vi "ChangeIndicator_RT.vi"(0 "Input":variant) -> (6 "Change":bool=TRUE)   [LabVIEW 2015, in "ECS-RT.lvlib"]
uses:
  ECS-RT.lvlib
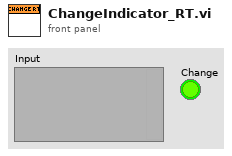
[diagram p1: front panel]
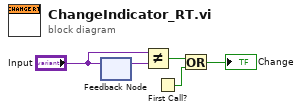
[diagram p0: block diagram]
diagram:
  n1 = feedback-in #1("Input") -> ()
  n2 = feedback #1() -> (w5:variant)  [unwired: 1 in]
  n3 = Not Equal?(x="Input", y=w5) -> (x != y?=w1:bool)
  n4 = First Call?() -> (First Call?: T/F=w2:bool)
  n5 = Or(x=w1, y=w2) -> (x .or. y?=→"Change":bool)
